vi "Close Accelerometer.vi"(8 "error in (no error)":errorcluster, 11 "Accelerometer":T1) -> (0 "error out":errorcluster)   [LabVIEW 2012]
doc: "Use this template to build a VI to use as a subVI."
uses:
  Accelerometer.ctl
  <vilib>/ni845x/ni845x.llb/ni845xControl.ctl
  <vilib>/ni845x/ni845x.llb/ni845xI2cConfiguration.ctl
  <vilib>/ni845x/ni845x.llb/NI-845x I2C Close Configuration Reference.vi
  <vilib>/ni845x/ni845x.llb/NI-845x Close Device Reference.vi
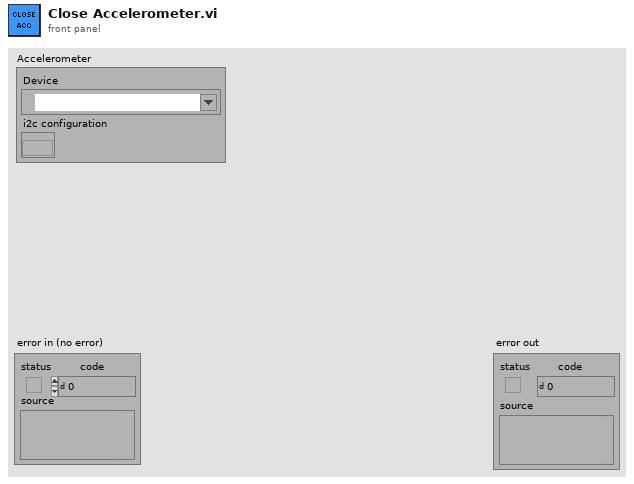
[diagram p1: front panel]
types:
  T1 = typedef "Accelerometer.ctl" = cluster{"Device":T2, "i2c configuration":T3}
  T2 = typedef "ni845xControl.ctl" = refnum<k21>
  T3 = typedef "ni845xI2cConfiguration.ctl" = refnum<k20>
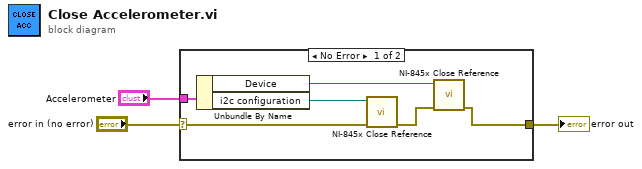
[diagram p0: block diagram]
diagram:
  n1 = case shown="No Error" "error in (no error)" {
    selector: "error in (no error)" -> [w7 w10]
    tunnel: [w4 w10] -> w2
    tunnel: "Accelerometer" -> [w9 _]
    frame No Error {
      n2 = Unbundle By Name(w9) -> ("Device"=w5:T2, "i2c configuration"=w8:T3)
      n3 = call-poly <vilib>:"NI-845x Close Reference.vi"("error in (no error)"=w7, "i2c configuration"=w8) -> ("error out"=w6:errorcluster)  [unwired: 9 in]
      n4 = call-poly <vilib>:"NI-845x Close Reference.vi"("error in (no error)"=w6, "device reference"=w5) -> ("error out"=w4:errorcluster)  [unwired: 9 in]
    }
    frame Error {
    }
  }
  "error out" <- w2
